vi "JKISM++ Start Async Call.vi"   [LabVIEW 2014, in "JKI-State-Machine-Plus.lvlib"]
uses:
  JKI-State-Machine-Plus.lvlib
  Templates/JKI State Machine ++ No Event Structure.vi
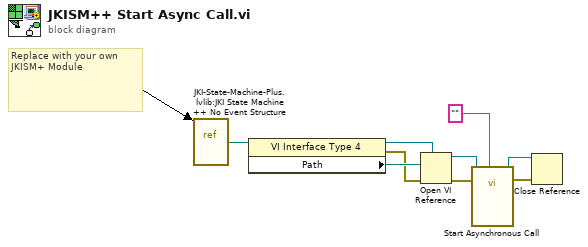
[diagram p0: block diagram]
diagram:
  # "Replace with your own JKISM+ Module"
  n1 = vi-ref "JKI-State-Machine-Plus.lvlib:JKI State Machine ++ No Event Structure.vi"() -> (w8:refnum<vi>)
  n2 = property class="VI Interface Type 4"(reference=w8) -> (reference out=w4:refnum<vi>, error out=w6:errorcluster, "Path"=w7:path)  [unwired: 1 in]
  n3 = Open VI Reference(type specifier VI Refnum (for type only)=w4, vi path=w7, error in (no error)=w6) -> (vi reference=w5:refnum<vi>, error out=w9:errorcluster)  [unwired: 3 in]
  n4 = call-by-ref "Start Asynchronous Call"(reference=w5, error in=w9, "Name(\"\" to use uuid)"="" ("Name(\"\" to use uuid)")) -> (reference out=w1:refnum<vi>, error out=w2:errorcluster)  [unwired: 11 in]
  n5 = Close Reference(reference=w1, error in (no error)=w2) -> ()  [unwired: 1 out]
